vi "Reporting_datetime.vi"() -> (3 "String":string)   [LabVIEW 2015]
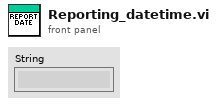
[diagram p1: front panel]
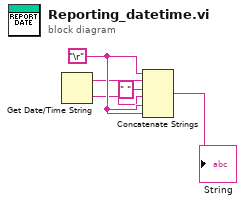
[diagram p0: block diagram]
diagram:
  w5 = "\r"
  n1 = Get Date/Time String() -> (date string=w1:string, time string=w3:string)  [unwired: 3 in]
  n2 = Concatenate Strings(w5, w1, " " ("string"), w3, w5, w5) -> (→"String":string)
